vi "About Panther Dashboard.vi"(8 "error in":errorcluster) -> (0 "error out":errorcluster)   [LabVIEW 2020, in "Panther Dashboard.lvlib"]
uses:
  Panther Dashboard.lvlib
  <vilib>/Platform/browser.llb/Open URL in Default Browser (string).vi
panel:
  in  "Website":bool
  out "Title":string
  in  "About DQMH":bool
  # "Maintained by: PantherLAB\nCLA Enrique Noé Arias\ninfo@pantherlab.com.mx"
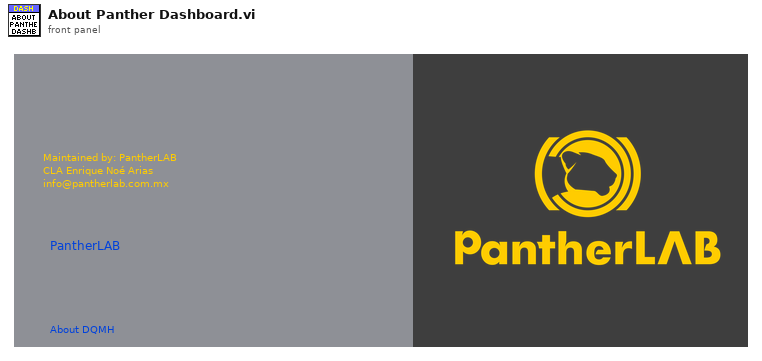
[diagram p1: front panel]
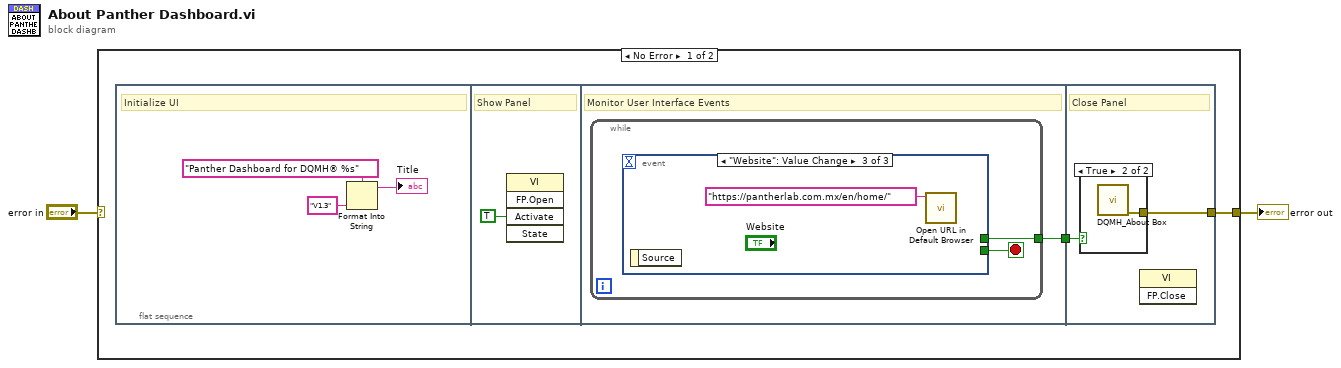
[diagram p0: block diagram]
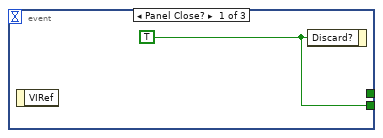
[diagram p2: hidden frame]
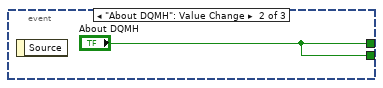
[diagram p3: hidden frame]
diagram:
  n1 = case shown="No Error" "error in" {
    selector: "error in" -> [_ w18]
    tunnel: [w4 w18] -> w1
    frame No Error {
      n2 = flat-sequence {
        tunnel: [w9] -> w3
        tunnel: w3 -> [w15]
        tunnel: [w16] -> w4
        frame #0 {
          # "Initialize UI"
          n3 = Format Into String(format string="Panther Dashboard for DQMH® %s" ("String"), "V1.3" ("input 1")) -> (resulting string=→"Title":string)  [unwired: 2 in, 1 out]
        }
        frame #1 {
          # "Show Panel"
          n4 = invoke class="VI" method="FP.Open"("Activate"=TRUE ("Activate?")) -> ()  [unwired: 4 in, 5 out]
        }
        frame #2 {
          # "Monitor User Interface Events"
          n5 = while {
            tunnel: [w10] -> w9
            stop <- w11 stop-if-true
            n6 = event shown="[2] \"Website\": Value Change" {
              selector: _ -> [_ _ _]
              dyn-events: _ -> [_ _ _]
              timeout: _ -> [_ _ _]
              tunnel: [w12 "About DQMH" _] -> w11
              tunnel: [_ "About DQMH" _] -> w10
              event Panel Close? {
                w12 = TRUE ("Discard?")
                n7 = event-data() -> ()  [unwired: 1 in, 1 out]
                n8 = event-data("Discard?"=w12) -> ()  [unwired: 1 in, 1 out]
              }
              event "About DQMH": Value Change {
                n9 = event-data() -> ()  [unwired: 1 in, 1 out]
              }
              event "Website": Value Change {
                n10 = event-data() -> ()  [unwired: 1 in, 1 out]
                n11 = call-poly <vilib>:"Open URL in Default Browser.vi"("URL"="https://pantherlab.com.mx/en/home/") -> ()  [unwired: 5 in, 2 out]
              }
            }
          }
        }
        frame #3 {
          # "Close Panel"
          n12 = case shown="True" w15 {
            tunnel: [_ w17] -> w16
            frame False {
            }
            frame True {
              n13 = call <vilib>:"DQMH_About Box.vi"() -> ("error out"=w17:errorcluster)  [unwired: 11 in]
            }
          }
          n14 = invoke class="VI" method="FP.Close"() -> ()  [unwired: 3 in, 3 out]
        }
      }
    }
    frame Error {
    }
  }
  "error out" <- w1
